vi "Int Write.vi"(5 "Data Block #":u16, 7 "Memory Area":T1, 8 "error in (no error)":errorcluster, 9 "Value":i16, 10 "Start Address":u32, 11 "S7 in":refnum<class "S7NetCom.lvclass">) -> (0 "error out":errorcluster, 3 "S7 out":refnum<class "S7NetCom.lvclass">)   [LabVIEW 2019]
uses:
  <vilib>/Hampel Software Engineering/S7NetCom/Source/S7NetCom.lvclass
  <vilib>/Hampel Software Engineering/S7NetCom/Source/Controls/S7_Memory_Area.ctl
  1af8ce59-7fb2-467f-9904-dfa4643619d6.vi
  <vilib>/Hampel Software Engineering/S7NetCom/Source/API/Write Data - Int (Scalar).vi
  <vilib>/Hampel Software Engineering/S7NetCom/Source/API/Read Data - Int (Scalar).vi
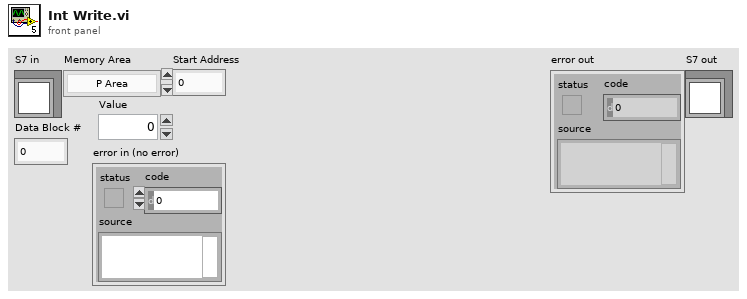
[diagram p1: front panel]
types:
  T1 = typedef "S7NetCom.lvlib/S7NetCom.lvclass/S7_Memory_Area.ctl" = enum8{"P Area", "I Area", "O Area", "M Area", "DB Area", "Counter", "Timer"}
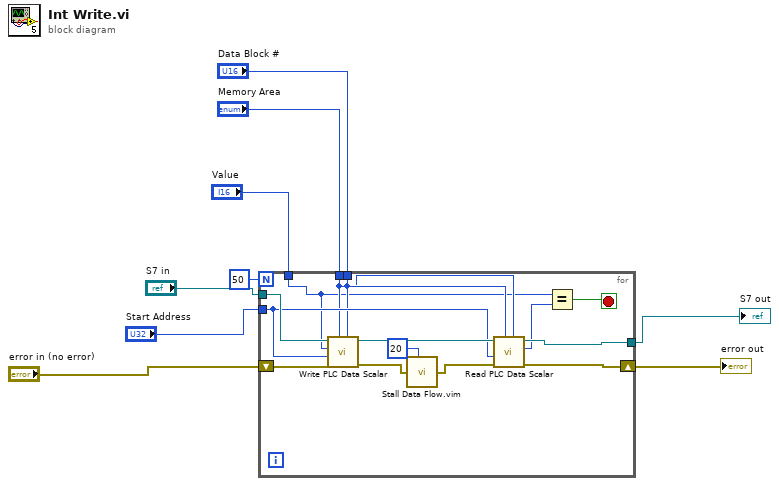
[diagram p0: block diagram]
diagram:
  n1 = for {
    N: 50 -> [_]
    tunnel: "Start Address" -> [w20]
    tunnel: "Memory Area" -> [w19]
    tunnel: "Data Block #" -> [w18]
    tunnel: "Value" -> [w10]
    shift-right: [w17] -> w3
    shift-left: "error in (no error)" -> [w22]
    tunnel: "S7 in" -> [w23]
    tunnel: [w16] -> w2
    stop <- w12 stop-if-true
    n2 = call-poly <vilib>:"Write PLC Data Scalar.vi"("Data Block #"=w18, "Memory Area"=w19, "error in (no error)"=w22, "Start Address"=w20, "Value"=w10, "S7 in"=w23) -> ("error out"=w15:errorcluster, "S7 out"=w21:refnum<class "S7NetCom.lvclass">)  [unwired: 4 in]
    n3 = call "Stall Data Flow.vim"("value in"=w15, "milliseconds to wait"=u32 20) -> ("value out"=w14:errorcluster)  [unwired: 1 out]
    n4 = call-poly <vilib>:"Read PLC Data Scalar.vi"("Data Block #"=w18, "Memory Area"=w19, "error in (no error)"=w14, "Start Address"=w20, "S7 in"=w21) -> ("error out"=w17:errorcluster, "Int Value"=w11:i16, "S7 out"=w16:refnum<class "S7NetCom.lvclass">)  [unwired: 4 in]
    n5 = Equal?(x=w10, y=w11) -> (x = y?=w12:bool)
  }
  "error out" <- w3
  "S7 out" <- w2
